vi "AverageVoltageNEW.vi"() -> ()   [LabVIEW 2020]
uses:
  <vilib>/Analysis/baseanly.llb/Mean (DBL).vi
  <vilib>/Analysis/NI_AALBase.lvlib
panel:
  out "Average Voltage Indicator":dbl
  in  "Average Time(s) Control":dbl
  in  "stop":bool
  out "Input Signal Graph":dynamicdata(graph)
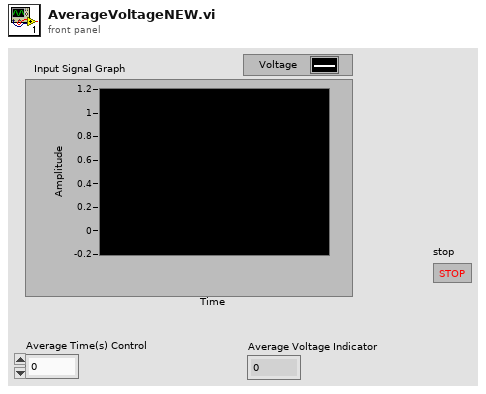
[diagram p1: front panel]
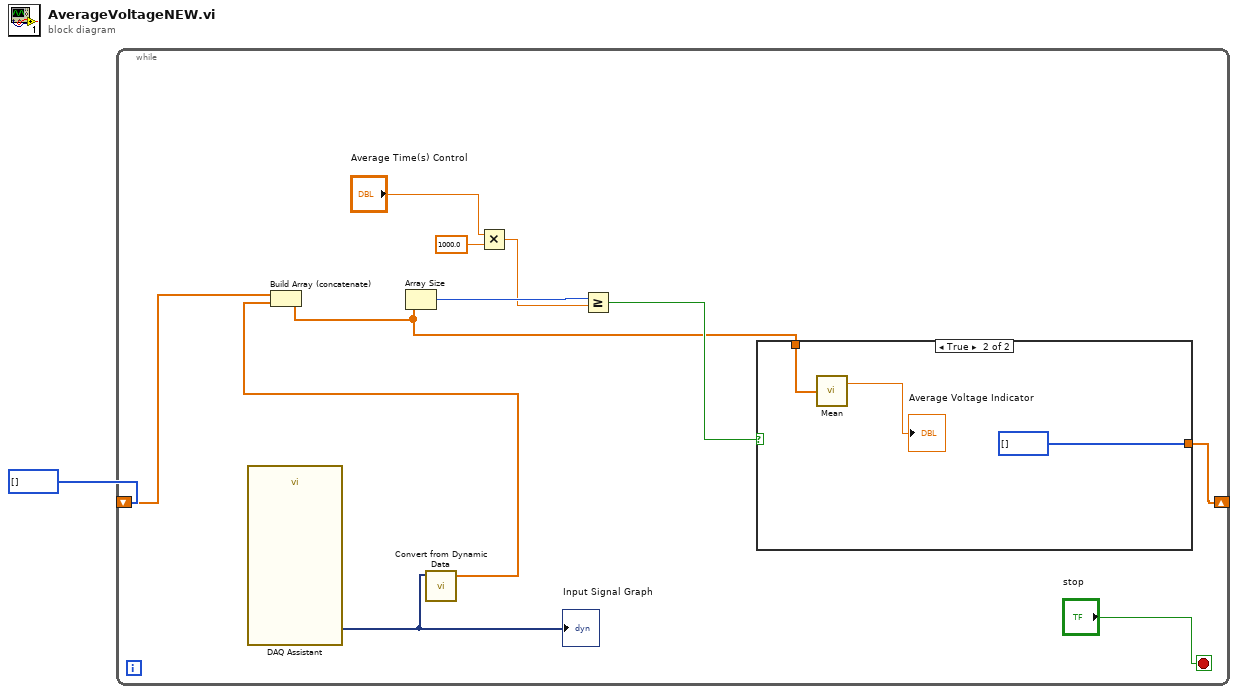
[diagram p0: block diagram]
diagram:
  n1 = while {
    shift-right: [w8] -> _
    shift-left: i32[] [] -> [w11]
    stop <- "stop" stop-if-true
    n2 = call "DAQ Assistant"() -> ("data"=w3:dynamicdata)  [unwired: 16 in, 3 out]
    "Input Signal Graph" <- w3
    n3 = call "Convert from Dynamic Data"("Dynamic Data Type"=w3) -> ("Array"=w2:dbl[])  [unwired: 3 in]
    n4 = Build Array (concatenate)(w11, w2) -> (w7:dbl[])
    n5 = Array Size(array=w7) -> (size(s)=w10:i32)
    n6 = Multiply(x="Average Time(s) Control", y=1000.0) -> (x*y=w4:dbl)
    n7 = Greater Or Equal?(x=w10, y=w4) -> (x >= y?=w9:bool)
    n8 = case shown="True" w9 {
      tunnel: w7 -> [w13 w16]
      tunnel: [w13 i32[] []] -> w8
      frame False {
      }
      frame True {
        n9 = call-poly <vilib>:"Mean.vi"("X"=w16) -> ("mean"=→"Average Voltage Indicator":dbl)  [unwired: 1 out]
      }
    }
  }
